vi "RandFreeDirection.vi"(9 "Intended Dir":T1, 11 "View":i32[](array[numeric])) -> (1 "Free space?":bool=TRUE, 3 "Direction":T1)   [LabVIEW 2020, in "Atom.lvclass"]
uses:
  Atom.lvclass
  Type Defs/Direction Enum.ctl
  5e4ca600-df69-4609-8023-248aceda87af.vi
  Type Defs/SB Type Defs.lvlib
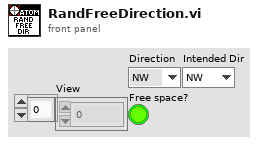
[diagram p1: front panel]
types:
  T1 = typedef "SB Type Defs.lvlib/Direction Enum.ctl" = enum16{"NW", "N", "NE", "E", "SE", "S", "SW", "W"}
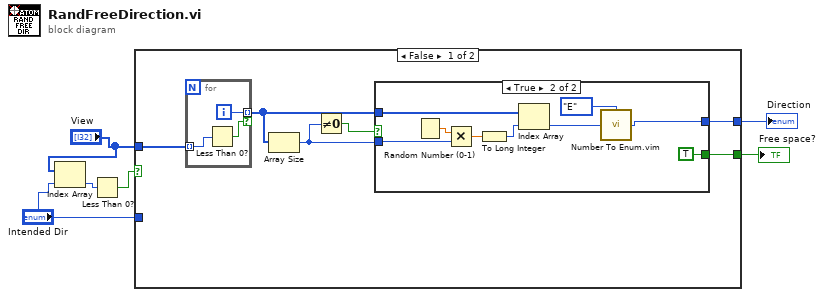
[diagram p0: block diagram]
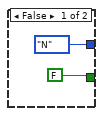
[diagram p2: hidden frame]
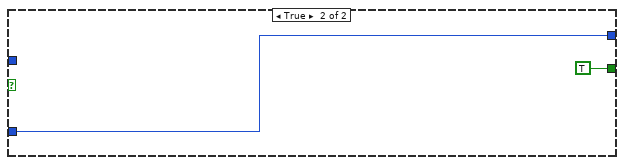
[diagram p3: hidden frame]
diagram:
  n1 = Index Array(array="View", index="Intended Dir") -> (element=w2:i32)
  n2 = Less Than 0?(x=w2) -> (x < 0?=w3:bool)
  n3 = case shown="False" w3 {
    tunnel: [w9 w28] -> w6
    tunnel: [w8 TRUE] -> w5
    tunnel: "View" -> [w7 _]
    tunnel: "Intended Dir" -> [_ w28]
    frame False {
      n4 = for {
        tunnel: [w26] -> w12 mode=indexing if=w25
        tunnel: w7 -> [w24] mode=indexing
        i -> [w26]
        n5 = Less Than 0?(x=w24) -> (x < 0?=w25:bool)
      }
      n6 = Array Size(array=w12) -> (size(s)=w11:i32)
      n7 = Not Equal To 0?(x=w11) -> (x != 0?=w10:bool)
      n8 = case shown="True" w10 {
        tunnel: w12 -> [_ w20]
        tunnel: w11 -> [_ w17]
        tunnel: [Direction_Enum."N" ("number as enum") w16] -> w9
        tunnel: [FALSE TRUE] -> w8
        frame False {
        }
        frame True {
          n9 = Random Number (0-1)() -> (number: 0 to 1=w22:dbl)
          n10 = Multiply(x=w22, y=w17) -> (x*y=w21:dbl)
          n11 = To Long Integer(number=w21) -> (32bit integer=w19:i32)
          n12 = Index Array(array=w20, index=w19) -> (element=w18:i32)
          n13 = call "Number To Enum.vim"("number"=w18, "enum type"=Direction_Enum."E" ("Direction")) -> ("number as enum"=w16:T1)
        }
      }
    }
    frame True {
    }
  }
  "Direction" <- w6
  "Free space?" <- w5
